vi "LabVIEW Environments Installed (Win10).vi"() -> (1 "Current LabVIEW x64 Index":i32, 2 "Current LabVIEW x86 Index":i32, 3 "LabVIEW Applications Installed":T1[](array[typedef]))   [LabVIEW 2020]
doc: "Created by Ryan Pacini"
uses:
  typedefs/LabViewApplication--cluster.ctl
  <vilib>/registry/registry.llb/Registry RtKey.ctl
  <vilib>/registry/registry.llb/Registry SAM.ctl
  <vilib>/registry/registry.llb/Registry View.ctl
  <vilib>/registry/registry.llb/Read Registry Value Simple STR.vi
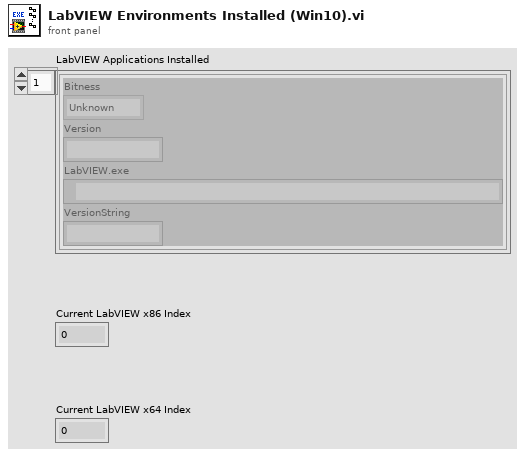
[diagram p1: front panel]
types:
  T1 = typedef "LabViewApplication--cluster.ctl" = cluster{"Bitness":enum8{"Unknown", "x86", "x64"}, "Version":string, "LabVIEW.exe":path, "VersionString":string}
  T2 = typedef "Registry View.ctl" = u16
  T3 = typedef "Registry SAM.ctl" = enum32{"KEY_QUERY_VALUE", "KEY_SET_VALUE", "KEY_CREATE_SUB_KEY", "KEY_ENUMERATE_SUB_KEYS", "KEY_NOTIFY", "KEY_CREATE_LINK", "KEY_READ", "KEY_WRITE", "KEY_ALL_ACCESS", "KEY_READ | KEY_WRITE"}
  T4 = typedef "Registry RtKey.ctl" = enum32{"HKEY_CLASSES_ROOT", "HKEY_CURRENT_USER", "HKEY_LOCAL_MACHINE", "HKEY_USERS", "HKEY_PERFORMANCE_DATA", "HKEY_CURRENT_CONFIG", "HKEY_DYN_DATA"}
  T5 = enum16{"open", "replace", "create", "open or create", "replace or create", "replace or create with confirmation"}
  T6 = typedef "Registry refnum.ctl" = refnum<k1>
  T7 = cluster{"numSubKeys":i32, "maxSubKeyLen":i32, "maxSubKeyClassLen":i32}
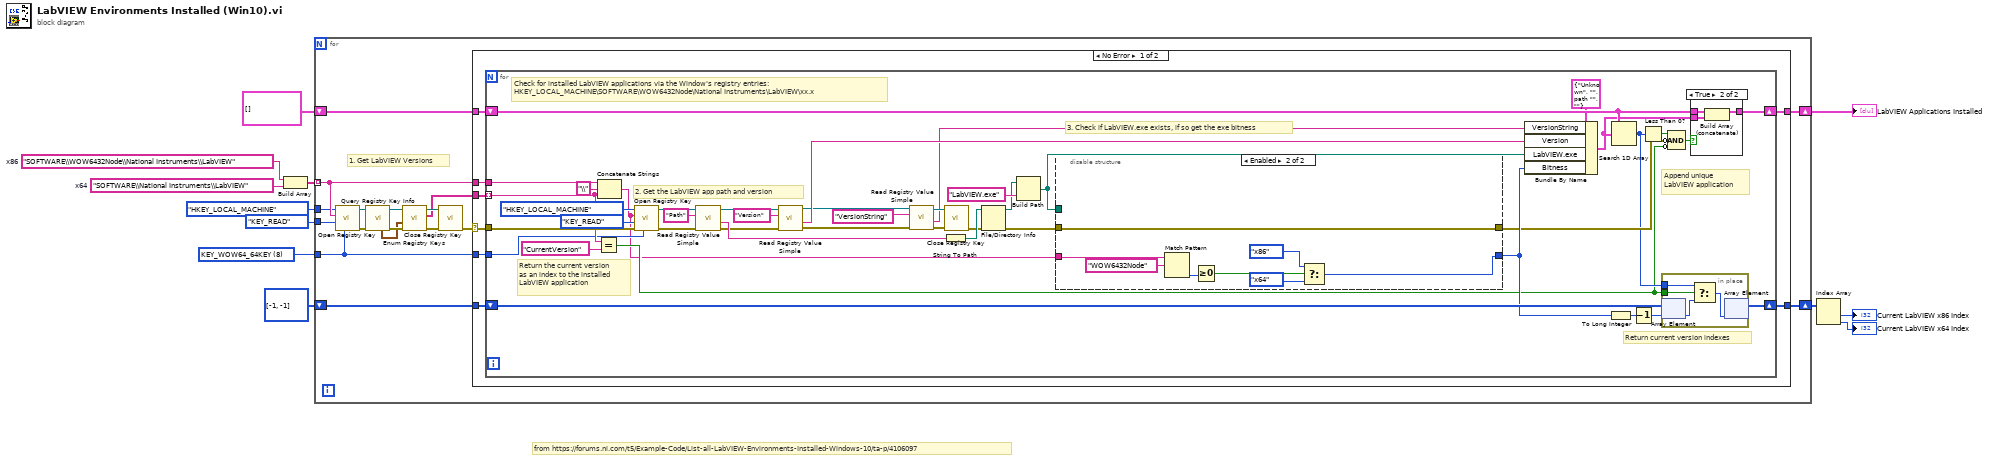
[diagram p0: block diagram]
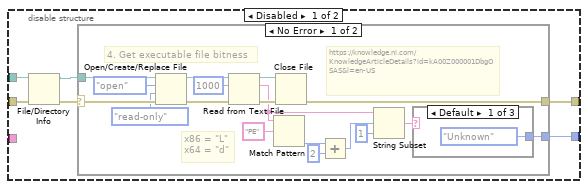
[diagram p2: hidden frame]
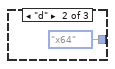
[diagram p3: hidden frame]
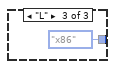
[diagram p4: hidden frame]
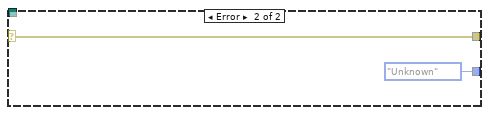
[diagram p5: hidden frame]
diagram:
  w1 = T2 8 items=["Default"=0, "KEY_WOW64_64KEY"=8, "KEY_WOW64_32KEY"=9] ("registry view")
  w5 = "SOFTWARE\\National Instruments\\LabVIEW"  # x64
  w12 = "SOFTWARE\\WOW6432Node\\National Instruments\\LabVIEW"  # x86
  # "from https://forums.ni.com/t5/Example-Code/List-all-LabVIEW-Environments-Installed-Windows-10/ta-p/4106097"
  n1 = Build Array(w12, w5) -> (w6:string[])
  n2 = for {
    tunnel: w6 -> [w21] mode=indexing
    shift-right: [w17] -> w9
    shift-left: T1[] [] ("LabVIEW Applications Installed") -> [w18]
    shift-right: [w19] -> w11
    shift-left: i32[] [-1, -1] ("index of element") -> [w16]
    tunnel: Registry_RtKey."HKEY_LOCAL_MACHINE" ("root key (HKEY_LOCAL_MACHINE)") -> [w15]
    tunnel: Registry_SAM."KEY_READ" ("security access mask (KEY_READ | KEY_WRITE)") -> [w14]
    tunnel: w1 -> [w13]
    # "1. Get LabVIEW Versions"
    n3 = call <vilib>:"Open Registry Key.vi"("registry view"=w13, "security access mask (KEY_READ | KEY_WRITE)"=w14, "subkey"=w21, "root key (HKEY_LOCAL_MACHINE)"=w15) -> ("error out"=w27:errorcluster, "refnum out"=w28:T6)  [unwired: 6 in]
    n4 = call <vilib>:"Query Registry Key Info.vi"("error in (no error)"=w27, "refnum"=w28) -> ("error out"=w25:errorcluster, "refnum out"=w26:T6, "subkey info"=w24:T7)  [unwired: 5 in, 2 out]
    n5 = call <vilib>:"Enum Registry Keys.vi"("error in (no error)"=w25, "subkey info"=w24, "refnum"=w26) -> ("error out"=w29:errorcluster, "subkeys"=w20:string[], "refnum out"=w22:T6)  [unwired: 6 in]
    n6 = call <vilib>:"Close Registry Key.vi"("error in (no error)"=w29, "refnum"=w22) -> ("error out"=w23:errorcluster)  [unwired: 5 in]
    n7 = case shown="No Error" w23 {
      selector: w23 -> [w37 _]
      tunnel: w21 -> [w36 _]
      tunnel: w20 -> [w35 _]
      tunnel: [w34 w127] -> w17
      tunnel: [w33 w126] -> w19
      tunnel: w18 -> [w32 w127]
      tunnel: w16 -> [w31 w126]
      tunnel: w13 -> [w30 _]
      frame No Error {
        n8 = for {
          tunnel: w36 -> [w74]
          tunnel: w35 -> [w49] mode=indexing
          tunnel: w37 -> [w79]
          shift-right: [w70] -> w34
          shift-left: w32 -> [w71]
          shift-right: [w59] -> w33
          shift-left: w31 -> [w60]
          tunnel: w30 -> [w46]
          # "Return the current version\nas an index to the installed\nLabVIEW application"
          # "Append unique\nLabVIEW application"
          # "Check for installed LabVIEW applications via the Window's registry entries:\nHKEY_LOCAL_MACHINE\\SOFTWARE\\WOW6432Node\\National Instruments\\LabVIEW\\xx.x"
          # "Return current version indexes"
          # "3. Check if LabVIEW.exe exists, if so get the exe bitness"
          # "2. Get the LabVIEW app path and version"
          n9 = Equal?(x=w49, y="CurrentVersion" ("x")) -> (x = y?=w48:bool)
          n10 = Concatenate Strings(w74, "\\" ("string"), w49) -> (w38:string)
          n11 = call <vilib>:"Open Registry Key.vi"("registry view"=w46, "error in (no error)"=w79, "security access mask (KEY_READ | KEY_WRITE)"=Registry_SAM."KEY_READ", "subkey"=w38, "root key (HKEY_LOCAL_MACHINE)"=Registry_RtKey."HKEY_LOCAL_MACHINE") -> ("error out"=w78:errorcluster, "refnum out"=w77:T6)  [unwired: 5 in]
          n12 = call-poly <vilib>:"Read Registry Value Simple.vi"("error in (no error)"=w78, "value"="Path", "refnum"=w77) -> ("error out"=w56:errorcluster, "String/Binary data"=w61:string, "refnum out"=w52:T6)  [unwired: 3 in, 1 out]
          n13 = call-poly <vilib>:"Read Registry Value Simple.vi"("error in (no error)"=w56, "value"="Version", "refnum"=w52) -> ("error out"=w43:errorcluster, "String/Binary data"=w50:string, "refnum out"=w42:T6)  [unwired: 3 in, 1 out]
          n14 = call-poly <vilib>:"Read Registry Value Simple.vi"("error in (no error)"=w43, "value"="VersionString", "refnum"=w42) -> ("error out"=w44:errorcluster, "String/Binary data"=w39:string, "refnum out"=w41:T6)  [unwired: 3 in, 1 out]
          n15 = String To Path(string=w61) -> (path=w76:path)
          n16 = call <vilib>:"Close Registry Key.vi"("error in (no error)"=w44, "refnum"=w41) -> ("error out"=w72:errorcluster)  [unwired: 5 in]
          n17 = File/Directory Info(path=w76, error in=w72) -> (path out=w68:path, error out=w67:errorcluster)  [unwired: 5 out]
          n18 = Build Path(base path=w68, name or relative path="LabVIEW.exe") -> (appended path=w47:path)
          n19 = disable-structure shown="Enabled" {
            disable-tunnel: w67 -> [w86 w117]
            disable-tunnel: [w84 w112] -> w58
            disable-tunnel: [w83 w117] -> w55
            disable-tunnel: w47 -> [w82 _]
            disable-tunnel: w38 -> [_ w115]
            frame Disabled {
              n20 = File/Directory Info(path=w82, error in=w86) -> (path out=w81:path, error out=w85:errorcluster)  [unwired: 5 out]
              n21 = case shown="No Error" w85 {
                selector: w85 -> [w104 w109]
                tunnel: [w87 enum8{"Unknown", "x86", "x64"}."Unknown" ("Bitness")] -> w84
                tunnel: [w103 w109] -> w83
                tunnel: w81 -> [w102 _]
                frame No Error {
                  # "x86 = \"L\"\nx64 = \"d\""
                  # "4. Get executable file bitness"
                  # "https://knowledge.ni.com/KnowledgeArticleDetails?id=kA00Z000001DbgOSAS&l=en-US"
                  n22 = Open/Create/Replace File(file path (use dialog)=w102, error in=w104, operation (0:open)=T5."open", access (0:read/write)=enum16{"read/write", "read-only", "write-only"}."read-only") -> (refnum out=w101:refnum<file>, error out=w100:errorcluster)  [unwired: 2 in, 1 out]
                  n23 = Read from Text File(file (use dialog)=w101, count=1000, error in=w100) -> (refnum out=w98:refnum<file>, text=w93:string, error out=w99:errorcluster)  [unwired: 1 in, 1 out]
                  n24 = Match Pattern(string=w93, regular expression="PE") -> (offset past match=w95:i32)  [unwired: 1 in, 3 out]
                  n25 = Close File(refnum=w98, error in=w99) -> (error out=w103:errorcluster)  [unwired: 1 out]
                  n26 = Add(x=w95, y=2) -> (x+y=w92:i32)
                  n27 = String Subset(string=w93, offset (0)=w92, length (rest)=1 ("length (rest)")) -> (substring=w88:string)
                  n28 = case shown="Default" w88 {
                    tunnel: [enum8{"Unknown", "x86", "x64"}."Unknown" ("Bitness") enum8{"Unknown", "x86", "x64"}."x64" ("Bitness") enum8{"Unknown", "x86", "x64"}."x86" ("Bitness")] -> w87
                    frame Default {
                    }
                    frame "d" {
                    }
                    frame "L" {
                    }
                  }
                }
                frame Error {
                }
              }
            }
            frame Enabled {
              n29 = Match Pattern(string=w115, regular expression="WOW6432Node") -> (offset past match=w116:i32)  [unwired: 1 in, 3 out]
              n30 = Greater Or Equal To 0?(x=w116) -> (x >= 0?=w113:bool)
              n31 = Select(t=enum8{"Unknown", "x86", "x64"}."x86" ("Bitness"), s=w113, f=enum8{"Unknown", "x86", "x64"}."x64" ("Bitness")) -> (s? t:f=w112:enum8{"Unknown", "x86", "x64"})
            }
          }
          n32 = Bundle By Name(cluster=T1 {"Bitness"=enum."Unknown", "Version"="", "LabVIEW.exe"=path "", "VersionString"=""} ("LabVIEW Application"), "VersionString"=w39, "Version"=w50, "LabVIEW.exe"=w47, "Bitness"=w58) -> (w64:T1)
          n33 = To Long Integer(number=w58) -> (32bit integer=w57:i32)
          n34 = Search 1D Array(1D array=w71, element=w64) -> (index of element=w54:i32)  [unwired: 1 in]
          n35 = Decrement(x=w57) -> (x-1=w53:i32)
          n36 = Less Than 0?(x=w54) -> (x < 0?=w66:bool)
          n37 = in-place {
            in-place-border: w54 -> [w121]
            in-place-border: w48 -> [w120]
            n38 = in-place-array #1(w60, w53) -> (w119:i32)
            n39 = Select(t=w121, s=w120, f=w119) -> (s? t:f=w118:i32)
            n40 = in-place-array #1(w118) -> (w59:i32[])  [unwired: 1 out]
          }
          n41 = Compound Arithmetic op=AND(w66, invert w55, invert w48) -> (w65:bool)
          n42 = case shown="True" w65 {
            tunnel: w71 -> [w122 w125]
            tunnel: w64 -> [_ w124]
            tunnel: [w122 w123] -> w70
            frame False {
            }
            frame True {
              n43 = Build Array (concatenate)(w125, w124) -> (w123:T1[])
            }
          }
        }
      }
      frame Error {
      }
    }
  }
  "LabVIEW Applications Installed" <- w9
  n44 = Index Array(array=w11) -> (element #1=→"Current LabVIEW x86 Index":i32, element #2=→"Current LabVIEW x64 Index":i32)  [unwired: 2 in]
